vi "Displacement.vi"   [LabVIEW 2018]
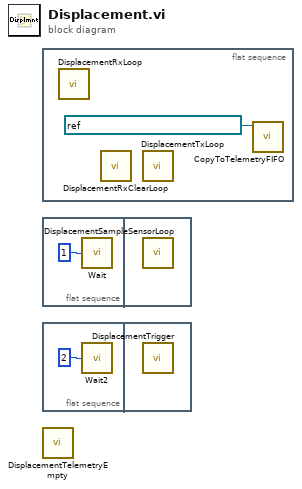
[diagram p0: block diagram]
diagram:
  n1 = flat-sequence {
    frame #0 {
      n2 = call "DisplacementRxLoop.vi"() -> ()  [unwired: 12 in]
      n3 = call "DisplacementRxClearLoop.vi"() -> ()  [unwired: 12 in]
      n4 = call "DisplacementTxLoop.vi"() -> ()  [unwired: 12 in]
      n5 = call "CopyToTelemetryFIFO.vi"("SourceFIFO"=refnum<k21> "DisplacementTelemetryFIFO") -> ()  [unwired: 11 in]
    }
  }
  n6 = flat-sequence {
    frame #0 {
      n7 = call "Wait"("Count(mSec)"=u8 1) -> ()  [unwired: 1 out]
    }
    frame #1 {
      n8 = call "DisplacementSampleSensorLoop.vi"() -> ()  [unwired: 12 in]
    }
  }
  n9 = flat-sequence {
    frame #0 {
      n10 = call "Wait2"("Count(mSec)"=u8 2) -> ()  [unwired: 1 out]
    }
    frame #1 {
      n11 = call "DisplacementTrigger.vi"() -> ()  [unwired: 12 in]
    }
  }
  n12 = call "DisplacementTelemetryEmpty.vi"() -> ()  [unwired: 12 in]
